vi "1.HMI.vi"() -> ()   [LabVIEW 2020]
uses:
  Control 6.ctl
  Niveles_tanques.vi
  Mezclador.vi
  Valvulas_On_Off.vi
  Bombas.vi
  Posicion_auto.vi
  Cepillo_Lavado.vi
  Cepilo_encerado.vi
  Ventilador.vi
  Estado_posicion_sensores.vi
  Motor_Banda_Transportadora.vi
  Posicion_limite_auto.vi
panel:
  out "Sensor 7":bool
  out "Cera 2":bool
  out "Cera 1":bool
  out "Jabon 3":bool
  out "Jabon 2":bool
  out "Jabon 1":bool
  out "Agua 3":bool
  out "Agua 2":bool
  out "Agua 1":bool
  out "Giro bomba cera":bool
  out "Giro bomba enjuague":bool
  out "Giro bomba jabon":bool
  out "Rueda 23":bool
  out "Rueda 22":bool
  out "Rueda 21":bool
  out "Rueda 20":bool
  out "Rueda 19":bool
  out "Rueda 18":bool
  out "Rueda 17":bool
  out "Rueda 16":bool
  out "Rueda 15":bool
  out "Rueda 14":bool
  out "Rueda 13":bool
  out "Rueda 12":bool
  out "Rueda 11":bool
  out "Rueda 10":bool
  out "Rueda 9":bool
  out "Rueda 8":bool
  out "Rueda 7":bool
  out "Rueda 6":bool
  out "Rueda 5":bool
  out "Rueda 4":bool
  out "Rueda 3":bool
  out "Rueda 2":bool
  out "Rueda 1":bool
  out "Motor Banda Transportadora":bool
  out "Sensor 6":bool
  out "Sensor 5":bool
  out "Sensor 4":bool
  out "Sensor 1":bool
  out "Sensor 3":bool
  out "Sensor 2":bool
  out "Ventilador":bool
  out "Cep_encer_2":T1
  out "Cep_Lavado 2":T1
  out "Cepillos encerado":bool
  out "Cepillos lavado":bool
  out "Bomba cera":bool
  out "Bomba jabon":bool
  out "Bomba enjuague":bool
  out "Valvula jabon":bool
  out "Valvula enjuague":bool
  out "Valvula cera":bool
  out "Valvula agua":bool
  out "Valvula Detergente":bool
  out "Cera":dbl(slide) scale=0.0..100.0
  out "Mezclador":bool
  out "Detergente":dbl(slide) scale=0.0..100.0
  out "Tanque de agua":dbl(slide)=100.0 scale=0.0..100.0
  out "Auto":bool
  out "Ring":u16(ring)
  out "Cep_Lavado 1":T1
  out "Cep_encer 1":T1
  # "1ra fase: entra el vehiculo a la bàscula que sensa el carro, se inicia la primera etapa\n1- Se mezcla agua con detergente neutro en un tanque, se mezcla.\n2- Avanza el vehiculo y a travès de unos inyectores se aplica el agua con el detergente hasta que llega\nal segundo sensor.\n3- Los rodillos con los cepillos empiezan a girar y continua el avance del automovil hasta el 3er sensor\n4- Inyectores con agua enjuagan el vehiculo hasta el cuarto sensor.\n5- Se aplica cera y luego pasa de nuevo por rodillos hasta el quinto sensor\n6- El vehiculo avanza y a la vez se seca con ventiladores hasta el sexto sensor"
  # "variables globales:\n-Mezclador\n-Niveles tanques\n-Valvulas\n-Bombas\n-Auto\n-Cepillo lavado\n-Cepillo encerado\nVentilador\n-Sensores\nmotor banda transportadora"
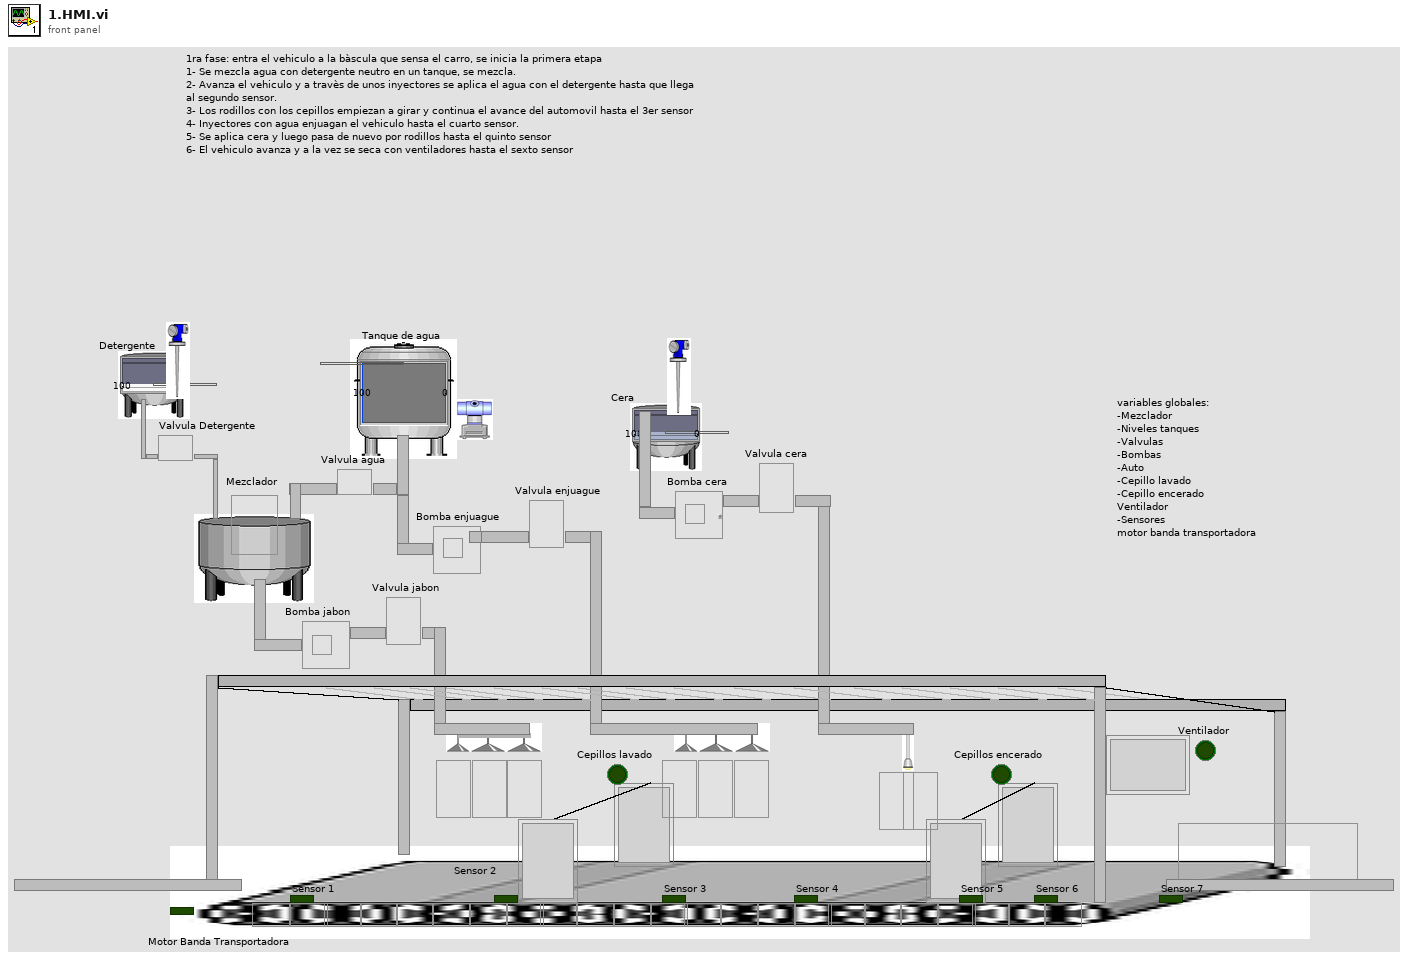
[diagram p1: front panel]
types:
  T1 = typedef "Control 6.ctl" = u16
  T2 = cluster{"Detergente":dbl, "Tanque de agua":dbl, "Cera":dbl}
  T3 = cluster{"Posicion limite izquierda":i32, "Posicion limite derecha":i32}
  T4 = cluster{"Valvula detergente":bool, "Valvula agua":bool, "Valvula  enjuague":bool, "Valvula  jabon":bool, "Valvula  cera":bool}
  T5 = cluster{"Bomba jabon":bool, "Bomba enjuague":bool, "Bomba cera":bool}
  T6 = cluster{"Posicion sensor 1":i32, "Posicion sensor 2":i32, "Posicion sensor 3":i32, "Posicion sensor 4":i32, "Posicion sensor 5":i32, "Posicion sensor 6":i32, "Estado sensor 1":bool, "Estado sensor 2":bool, "Estado sensor 3":bool, "Estado sensor 4":bool, "Estado sensor 5":bool, "Estado sensor 6":bool, "Posicion sensor 7":i32, "Estado sensor 7":bool}
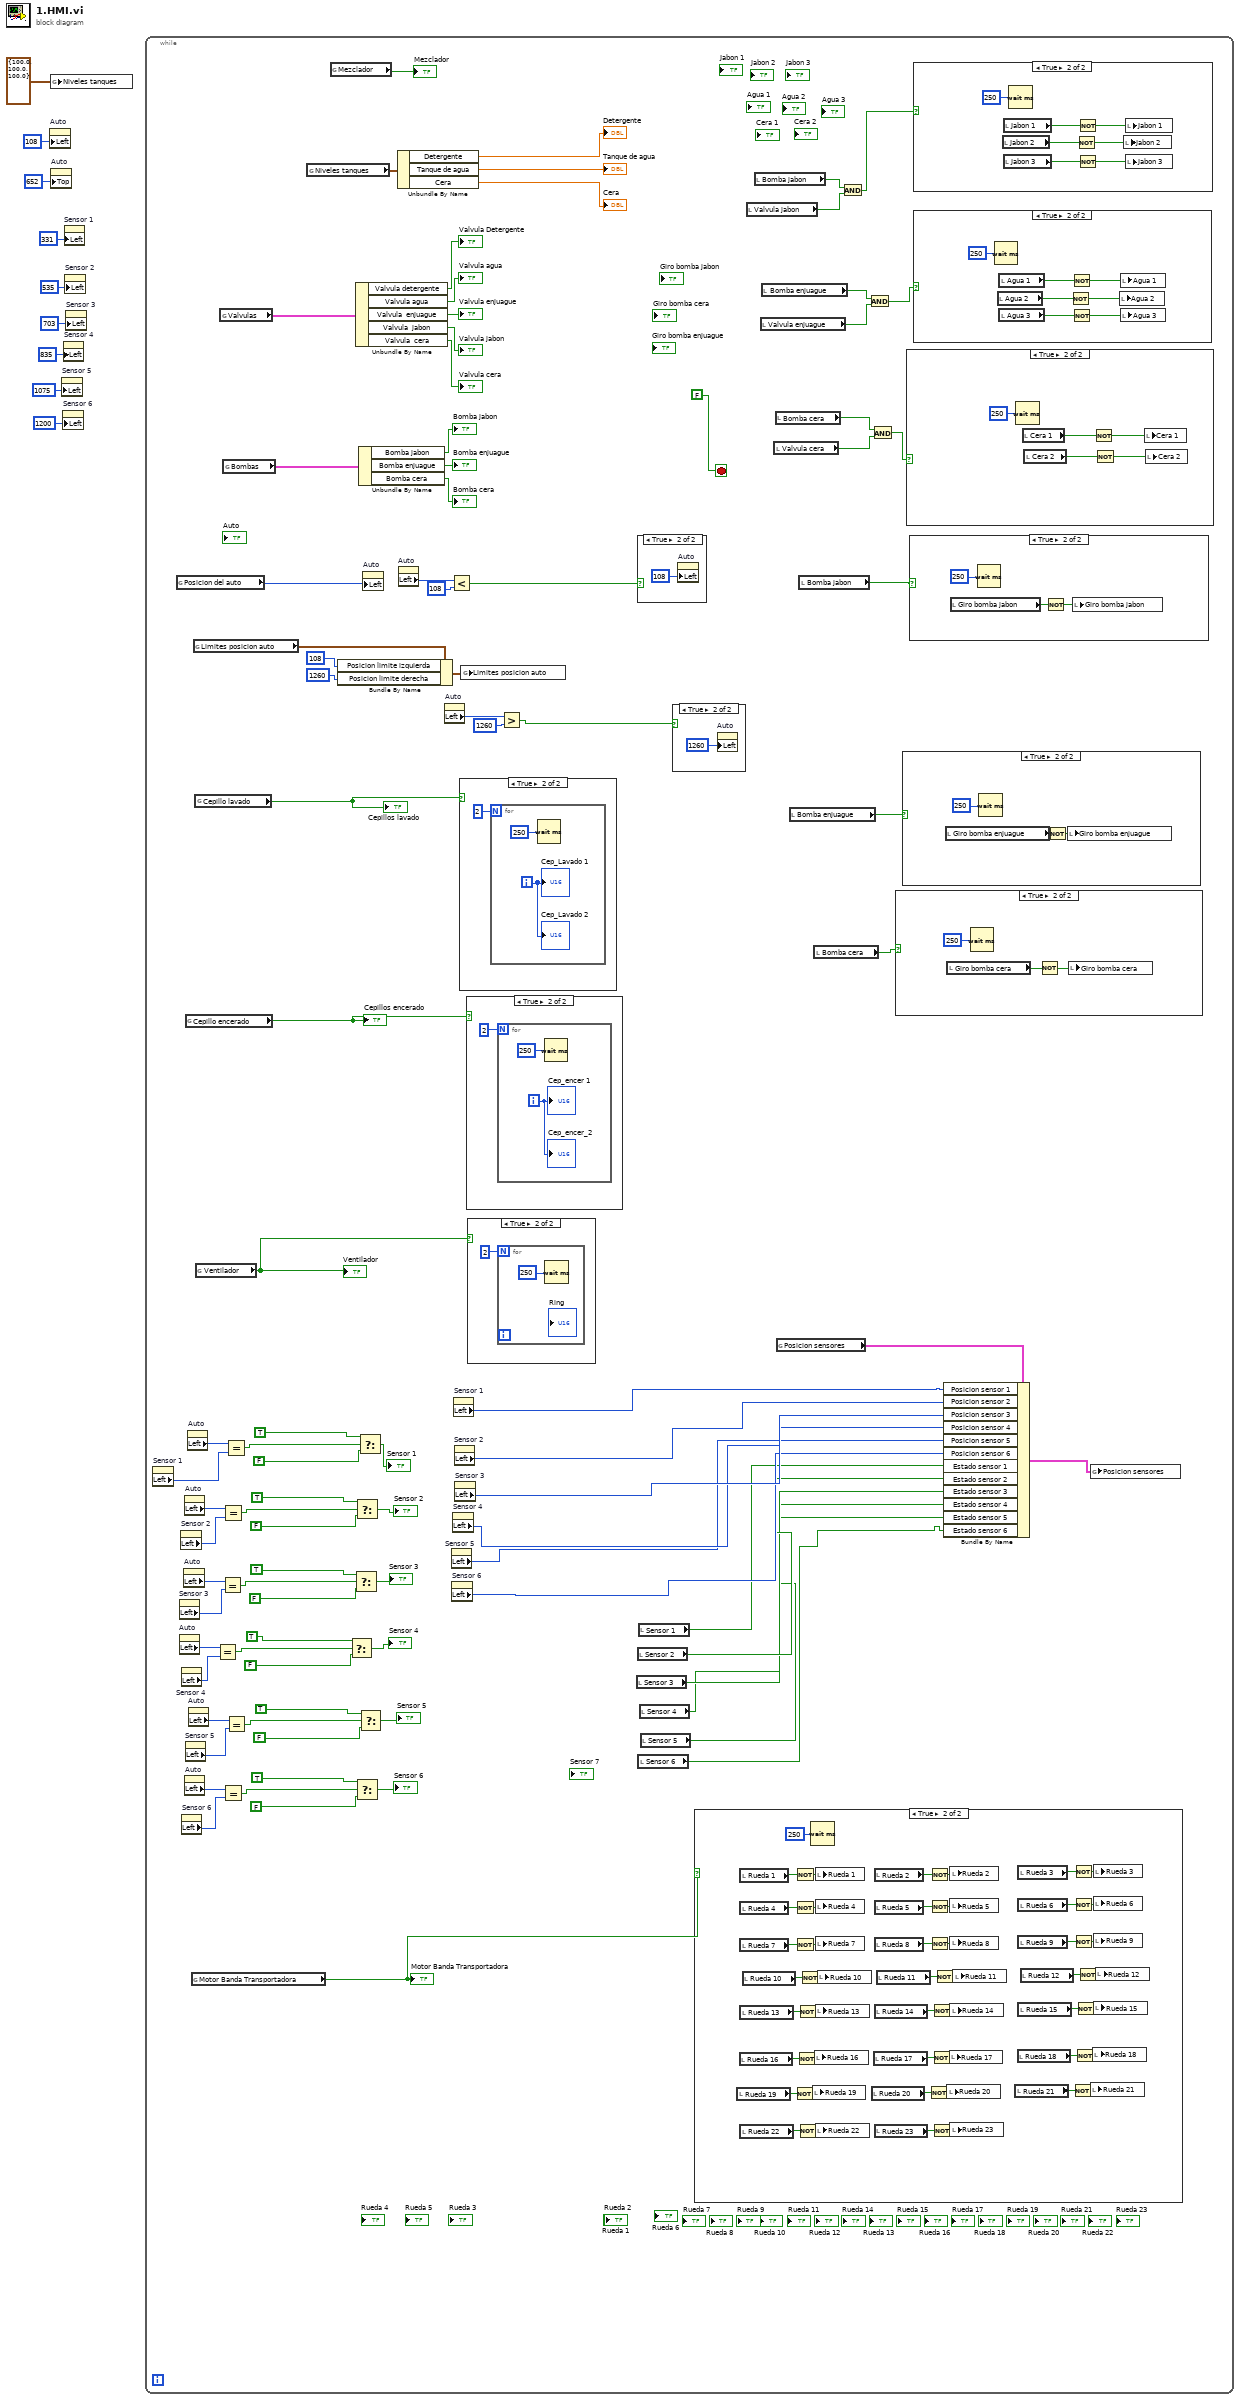
[diagram p0: block diagram]
diagram:
  n1 = property on="Auto" class="Bool (strict)"("Left"=108 ("Position:Left")) -> ()  [unwired: 2 in, 2 out]
  n2 = global write "Niveles_tanques.vi" "Niveles tanques"(T2 {"Detergente"=100.0, "Tanque de agua"=100.0, "Cera"=100.0} ("Niveles tanques")) -> ()
  n3 = property on="Auto" class="Bool (strict)"("Top"=652 ("Position:Top")) -> ()  [unwired: 2 in, 2 out]
  n4 = property on="Sensor 5" class="Bool (strict)"("Left"=1075 ("Position:Left")) -> ()  [unwired: 2 in, 2 out]
  n5 = property on="Sensor 6" class="Bool (strict)"("Left"=1200 ("Position:Left")) -> ()  [unwired: 2 in, 2 out]
  n6 = property on="Sensor 4" class="Bool (strict)"("Left"=835 ("Position:Left")) -> ()  [unwired: 2 in, 2 out]
  n7 = property on="Sensor 1" class="Bool (strict)"("Left"=331 ("Position:Left")) -> ()  [unwired: 2 in, 2 out]
  n8 = property on="Sensor 2" class="Bool (strict)"("Left"=535 ("Position:Left")) -> ()  [unwired: 2 in, 2 out]
  n9 = property on="Sensor 3" class="Bool (strict)"("Left"=703 ("Position:Left")) -> ()  [unwired: 2 in, 2 out]
  n10 = while {
    stop <- FALSE stop-if-true
    n11 = property on="Sensor 1" class="Bool (strict)"() -> ("Left"=w58:i32)  [unwired: 2 in, 2 out]
    n12 = global read "Posicion_auto.vi" "Posicion del auto"() -> (w80:i32)
    n13 = property on="Sensor 3" class="Bool (strict)"() -> ("Left"=w30:i32)  [unwired: 2 in, 2 out]
    n14 = property on="Auto" class="Bool (strict)"() -> ("Left"=w47:i32)  [unwired: 2 in, 2 out]
    n15 = property on="Sensor 2" class="Bool (strict)"() -> ("Left"=w31:i32)  [unwired: 2 in, 2 out]
    n16 = property on="Sensor 4" class="Bool (strict)"() -> ("Left"=w29:i32)  [unwired: 2 in, 2 out]
    n17 = property on="Sensor 6" class="Bool (strict)"() -> ("Left"=w27:i32)  [unwired: 2 in, 2 out]
    n18 = property on="Auto" class="Bool (strict)"() -> ("Left"=w50:i32)  [unwired: 2 in, 2 out]
    n19 = property on="Auto" class="Bool (strict)"() -> ("Left"=w55:i32)  [unwired: 2 in, 2 out]
    n20 = property on="Auto" class="Bool (strict)"() -> ("Left"=w39:i32)  [unwired: 2 in, 2 out]
    n21 = global read "Cepilo_encerado.vi" "Cepillo encerado"() -> (w78:bool)
    "Cepillos encerado" <- w78
    n22 = property on="Sensor 5" class="Bool (strict)"() -> ("Left"=w28:i32)  [unwired: 2 in, 2 out]
    n23 = property on="Auto" class="Bool (strict)"() -> ("Left"=w59:i32)  [unwired: 2 in, 2 out]
    n24 = property on="Auto" class="Bool (strict)"() -> ("Left"=w42:i32)  [unwired: 2 in, 2 out]
    n25 = global read "Motor_Banda_Transportadora.vi" "Motor Banda Transportadora"() -> (w26:bool)
    "Motor Banda Transportadora" <- w26
    n26 = global read "Posicion_limite_auto.vi" "Limites posicion auto"() -> (w13:T3)
    n27 = global read "Cepillo_Lavado.vi" "Cepillo lavado"() -> (w79:bool)
    "Cepillos lavado" <- w79
    n28 = global read "Ventilador.vi" "Ventilador"() -> (w77:bool)
    "Ventilador" <- w77
    n29 = Equal?(x=w47, y=w29) -> (x = y?=w48:bool)
    n30 = global read "Valvulas_On_Off.vi" "Valvulas"() -> (w97:T4)
    n31 = Equal?(x=w50, y=w30) -> (x = y?=w49:bool)
    n32 = Equal?(x=w55, y=w31) -> (x = y?=w56:bool)
    n33 = Equal?(x=w39, y=w27) -> (x = y?=w40:bool)
    n34 = global read "Bombas.vi" "Bombas"() -> (w90:T5)
    n35 = Equal?(x=w59, y=w58) -> (x = y?=w57:bool)
    n36 = Equal?(x=w42, y=w28) -> (x = y?=w41:bool)
    n37 = global read "Niveles_tanques.vi" "Niveles tanques"() -> (w101:T2)
    n38 = global read "Mezclador.vi" "Mezclador"() -> (→"Mezclador":bool)
    n39 = Bundle By Name(cluster=w13, "Posicion limite izquierda"=108, "Posicion limite derecha"=1260) -> (w12:T3)
    n40 = Select(t=TRUE, s=w48, f=FALSE) -> (s? t:f=→"Sensor 4":bool)
    n41 = Select(t=TRUE, s=w49, f=FALSE) -> (s? t:f=→"Sensor 3":bool)
    n42 = Select(t=TRUE, s=w56, f=FALSE) -> (s? t:f=→"Sensor 2":bool)
    n43 = Select(t=TRUE, s=w40, f=FALSE) -> (s? t:f=→"Sensor 6":bool)
    n44 = Unbundle By Name(w97) -> ("Valvula detergente"=→"Valvula Detergente":bool, "Valvula agua"=→"Valvula agua":bool, "Valvula  enjuague"=→"Valvula enjuague":bool, "Valvula  jabon"=→"Valvula jabon":bool, "Valvula  cera"=→"Valvula cera":bool)
    n45 = Select(t=TRUE, s=w57, f=FALSE) -> (s? t:f=→"Sensor 1":bool)
    n46 = Unbundle By Name(w90) -> ("Bomba jabon"=→"Bomba jabon":bool, "Bomba enjuague"=→"Bomba enjuague":bool, "Bomba cera"=→"Bomba cera":bool)
    n47 = Select(t=TRUE, s=w41, f=FALSE) -> (s? t:f=→"Sensor 5":bool)
    n48 = property on="Auto" class="Bool (strict)"("Left"=w80) -> ()  [unwired: 2 in, 2 out]
    n49 = Unbundle By Name(w101) -> ("Detergente"=→"Detergente":dbl, "Tanque de agua"=→"Tanque de agua":dbl, "Cera"=→"Cera":dbl)
    n50 = property on="Auto" class="Bool (strict)"() -> ("Left"=w86:i32)  [unwired: 2 in, 2 out]
    n51 = property on="Auto" class="Bool (strict)"() -> ("Left"=w85:i32)  [unwired: 2 in, 2 out]
    n52 = Less?(x=w86, y=108) -> (x < y?=w82:bool)
    n53 = property on="Sensor 5" class="Bool (strict)"() -> ("Left"=w71:i32)  [unwired: 2 in, 2 out]
    n54 = property on="Sensor 6" class="Bool (strict)"() -> ("Left"=w70:i32)  [unwired: 2 in, 2 out]
    n55 = property on="Sensor 4" class="Bool (strict)"() -> ("Left"=w72:i32)  [unwired: 2 in, 2 out]
    n56 = property on="Sensor 1" class="Bool (strict)"() -> ("Left"=w75:i32)  [unwired: 2 in, 2 out]
    n57 = property on="Sensor 2" class="Bool (strict)"() -> ("Left"=w74:i32)  [unwired: 2 in, 2 out]
    n58 = property on="Sensor 3" class="Bool (strict)"() -> ("Left"=w73:i32)  [unwired: 2 in, 2 out]
    n59 = case shown="True" w79 {
      frame False {
      }
      frame True {
        n60 = for {
          N: 2 -> [_]
          i -> [w185]
          n61 = Wait (ms)(milliseconds to wait=u32 250) -> ()  [unwired: 1 out]
          "Cep_Lavado 1" <- w185
          "Cep_Lavado 2" <- w185
        }
      }
    }
    n62 = global write "Posicion_limite_auto.vi" "Limites posicion auto"(w12) -> ()
    n63 = case shown="True" w78 {
      frame False {
      }
      frame True {
        n64 = for {
          N: 2 -> [_]
          i -> [w182]
          n65 = Wait (ms)(milliseconds to wait=u32 250) -> ()  [unwired: 1 out]
          "Cep_encer 1" <- w182
          "Cep_encer_2" <- w182
        }
      }
    }
    n66 = case shown="True" w77 {
      frame False {
      }
      frame True {
        n67 = for {
          N: 2 -> [_]
          n68 = Wait (ms)(milliseconds to wait=u32 250) -> ()  [unwired: 1 out]
        }
      }
    }
    n69 = Greater?(x=w85, y=1260) -> (0:w81:bool)
    n70 = local read "Sensor 3"() -> (w67:bool)
    n71 = local read "Sensor 2"() -> (w68:bool)
    n72 = case shown="True" w82 {
      frame False {
      }
      frame True {
        n73 = property on="Auto" class="Bool (strict)"("Left"=108 ("Position:Left")) -> ()  [unwired: 2 in, 2 out]
      }
    }
    n74 = local read "Sensor 6"() -> (w64:bool)
    n75 = local read "Sensor 1"() -> (w69:bool)
    n76 = local read "Sensor 4"() -> (w66:bool)
    n77 = local read "Sensor 5"() -> (w65:bool)
    n78 = case shown="True" w81 {
      frame False {
      }
      frame True {
        n79 = property on="Auto" class="Bool (strict)"("Left"=1260 ("Position:Left")) -> ()  [unwired: 2 in, 2 out]
      }
    }
    n80 = case shown="True" w26 {
      frame False {
      }
      frame True {
        n81 = local read "Rueda 19"() -> (w141:bool)
        n82 = local read "Rueda 16"() -> (w142:bool)
        n83 = local read "Rueda 1"() -> (w177:bool)
        n84 = local read "Rueda 4"() -> (w166:bool)
        n85 = local read "Rueda 7"() -> (w165:bool)
        n86 = local read "Rueda 13"() -> (w153:bool)
        n87 = local read "Rueda 22"() -> (w132:bool)
        n88 = local read "Rueda 10"() -> (w154:bool)
        n89 = Not(x=w141) -> (.not. x?=w140:bool)
        n90 = Not(x=w177) -> (.not. x?=w176:bool)
        n91 = Not(x=w166) -> (.not. x?=w167:bool)
        n92 = Not(x=w165) -> (.not. x?=w164:bool)
        n93 = Not(x=w142) -> (.not. x?=w143:bool)
        n94 = Not(x=w153) -> (.not. x?=w152:bool)
        n95 = Not(x=w132) -> (.not. x?=w133:bool)
        n96 = Not(x=w154) -> (.not. x?=w155:bool)
        n97 = Wait (ms)(milliseconds to wait=u32 250) -> ()  [unwired: 1 out]
        n98 = local write "Rueda 19"(w140) -> ()
        n99 = local write "Rueda 16"(w143) -> ()
        n100 = local write "Rueda 1"(w176) -> ()
        n101 = local write "Rueda 4"(w167) -> ()
        n102 = local write "Rueda 7"(w164) -> ()
        n103 = local write "Rueda 13"(w152) -> ()
        n104 = local write "Rueda 22"(w133) -> ()
        n105 = local write "Rueda 10"(w155) -> ()
        n106 = local read "Rueda 20"() -> (w138:bool)
        n107 = local read "Rueda 17"() -> (w145:bool)
        n108 = local read "Rueda 2"() -> (w174:bool)
        n109 = local read "Rueda 5"() -> (w169:bool)
        n110 = local read "Rueda 8"() -> (w162:bool)
        n111 = local read "Rueda 14"() -> (w150:bool)
        n112 = local read "Rueda 23"() -> (w135:bool)
        n113 = local read "Rueda 11"() -> (w157:bool)
        n114 = Not(x=w138) -> (.not. x?=w139:bool)
        n115 = Not(x=w174) -> (.not. x?=w175:bool)
        n116 = Not(x=w169) -> (.not. x?=w168:bool)
        n117 = Not(x=w162) -> (.not. x?=w163:bool)
        n118 = Not(x=w145) -> (.not. x?=w144:bool)
        n119 = Not(x=w150) -> (.not. x?=w151:bool)
        n120 = Not(x=w135) -> (.not. x?=w134:bool)
        n121 = Not(x=w157) -> (.not. x?=w156:bool)
        n122 = local write "Rueda 20"(w139) -> ()
        n123 = local write "Rueda 17"(w144) -> ()
        n124 = local write "Rueda 2"(w175) -> ()
        n125 = local write "Rueda 5"(w168) -> ()
        n126 = local write "Rueda 8"(w163) -> ()
        n127 = local write "Rueda 14"(w151) -> ()
        n128 = local write "Rueda 23"(w134) -> ()
        n129 = local write "Rueda 11"(w156) -> ()
        n130 = local read "Rueda 21"() -> (w137:bool)
        n131 = local read "Rueda 18"() -> (w146:bool)
        n132 = local read "Rueda 3"() -> (w173:bool)
        n133 = local read "Rueda 6"() -> (w170:bool)
        n134 = local read "Rueda 9"() -> (w161:bool)
        n135 = local read "Rueda 15"() -> (w149:bool)
        n136 = local read "Rueda 12"() -> (w158:bool)
        n137 = Not(x=w137) -> (.not. x?=w136:bool)
        n138 = Not(x=w173) -> (.not. x?=w172:bool)
        n139 = Not(x=w170) -> (.not. x?=w171:bool)
        n140 = Not(x=w161) -> (.not. x?=w160:bool)
        n141 = Not(x=w146) -> (.not. x?=w147:bool)
        n142 = Not(x=w149) -> (.not. x?=w148:bool)
        n143 = Not(x=w158) -> (.not. x?=w159:bool)
        n144 = local write "Rueda 21"(w136) -> ()
        n145 = local write "Rueda 18"(w147) -> ()
        n146 = local write "Rueda 3"(w172) -> ()
        n147 = local write "Rueda 6"(w171) -> ()
        n148 = local write "Rueda 9"(w160) -> ()
        n149 = local write "Rueda 15"(w148) -> ()
        n150 = local write "Rueda 12"(w159) -> ()
      }
    }
    n151 = local read "Valvula jabon"() -> (w21:bool)
    n152 = local read "Bomba jabon"() -> (w22:bool)
    n153 = local read "Valvula enjuague"() -> (w17:bool)
    n154 = local read "Bomba enjuague"() -> (w19:bool)
    n155 = local read "Valvula cera"() -> (w15:bool)
    n156 = local read "Bomba cera"() -> (w16:bool)
    n157 = global read "Estado_posicion_sensores.vi" "Posicion sensores"() -> (w76:T6)
    n158 = local read "Bomba enjuague"() -> (w23:bool)
    n159 = local read "Bomba jabon"() -> (w25:bool)
    n160 = local read "Bomba cera"() -> (w24:bool)
    n161 = And(x=w22, y=w21) -> (x .and. y?=w20:bool)
    n162 = And(x=w19, y=w17) -> (x .and. y?=w18:bool)
    n163 = And(x=w16, y=w15) -> (x .and. y?=w14:bool)
    n164 = case shown="True" w24 {
      frame False {
      }
      frame True {
        n165 = local read "Giro bomba cera"() -> (w124:bool)
        n166 = Wait (ms)(milliseconds to wait=u32 250) -> ()  [unwired: 1 out]
        n167 = Not(x=w124) -> (.not. x?=w123:bool)
        n168 = local write "Giro bomba cera"(w123) -> ()
      }
    }
    n169 = case shown="True" w23 {
      frame False {
      }
      frame True {
        n170 = local read "Giro bomba enjuague"() -> (w127:bool)
        n171 = Wait (ms)(milliseconds to wait=u32 250) -> ()  [unwired: 1 out]
        n172 = Not(x=w127) -> (.not. x?=w126:bool)
        n173 = local write "Giro bomba enjuague"(w126) -> ()
      }
    }
    n174 = case shown="True" w14 {
      frame False {
      }
      frame True {
        n175 = Wait (ms)(milliseconds to wait=u32 250) -> ()  [unwired: 1 out]
        n176 = local read "Cera 1"() -> (w107:bool)
        n177 = local read "Cera 2"() -> (w104:bool)
        n178 = Not(x=w107) -> (.not. x?=w106:bool)
        n179 = Not(x=w104) -> (.not. x?=w105:bool)
        n180 = local write "Cera 1"(w106) -> ()
        n181 = local write "Cera 2"(w105) -> ()
      }
    }
    n182 = case shown="True" w25 {
      frame False {
      }
      frame True {
        n183 = local read "Giro bomba jabon"() -> (w130:bool)
        n184 = Wait (ms)(milliseconds to wait=u32 250) -> ()  [unwired: 1 out]
        n185 = Not(x=w130) -> (.not. x?=w129:bool)
        n186 = local write "Giro bomba jabon"(w129) -> ()
      }
    }
    n187 = case shown="True" w20 {
      frame False {
      }
      frame True {
        n188 = local read "Jabon 2"() -> (w118:bool)
        n189 = local read "Jabon 1"() -> (w121:bool)
        n190 = local read "Jabon 3"() -> (w117:bool)
        n191 = Wait (ms)(milliseconds to wait=u32 250) -> ()  [unwired: 1 out]
        n192 = Not(x=w118) -> (.not. x?=w119:bool)
        n193 = Not(x=w121) -> (.not. x?=w120:bool)
        n194 = Not(x=w117) -> (.not. x?=w116:bool)
        n195 = local write "Jabon 2"(w119) -> ()
        n196 = local write "Jabon 1"(w120) -> ()
        n197 = local write "Jabon 3"(w116) -> ()
      }
    }
    n198 = case shown="True" w18 {
      frame False {
      }
      frame True {
        n199 = Wait (ms)(milliseconds to wait=u32 250) -> ()  [unwired: 1 out]
        n200 = local read "Agua 2"() -> (w111:bool)
        n201 = local read "Agua 1"() -> (w114:bool)
        n202 = local read "Agua 3"() -> (w110:bool)
        n203 = Not(x=w111) -> (.not. x?=w112:bool)
        n204 = Not(x=w114) -> (.not. x?=w113:bool)
        n205 = Not(x=w110) -> (.not. x?=w109:bool)
        n206 = local write "Agua 2"(w112) -> ()
        n207 = local write "Agua 1"(w113) -> ()
        n208 = local write "Agua 3"(w109) -> ()
      }
    }
    n209 = Bundle By Name(cluster=w76, "Posicion sensor 1"=w75, "Posicion sensor 2"=w74, "Posicion sensor 3"=w73, "Posicion sensor 4"=w72, "Posicion sensor 5"=w71, "Posicion sensor 6"=w70, "Estado sensor 1"=w69, "Estado sensor 2"=w68, "Estado sensor 3"=w67, "Estado sensor 4"=w66, "Estado sensor 5"=w65, "Estado sensor 6"=w64) -> (w63:T6)
    n210 = global write "Estado_posicion_sensores.vi" "Posicion sensores"(w63) -> ()
  }
